vi "Method 2.vi"(8 "error in (no error)":errorcluster, 11 "Interface 2 in":refnum<class "Interface 2.lvclass">) -> (0 "error out":errorcluster, 3 "Interface 2 out":refnum<class "Interface 2.lvclass">)   [LabVIEW 2021, in "Interface 2.lvclass"]
uses:
  Interface 2.lvclass
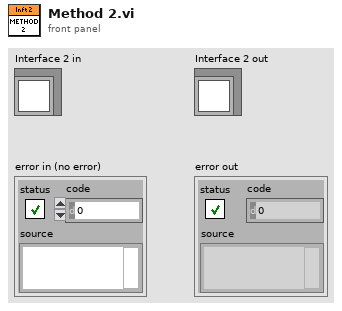
[diagram p1: front panel]
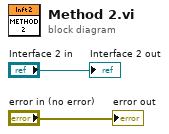
[diagram p0: block diagram]
diagram:
  "error out" <- "error in (no error)"
  "Interface 2 out" <- "Interface 2 in"
